vi "tm_preparecapture.vi"(8 "error in (no error)":errorcluster, 9 "Frames":i32, 10 "Capture mode":i32(ring) items=["Snap", "Sequence"], 11 "Handle in":u32) -> (0 "error out":errorcluster, 2 "Buffer":T1, 3 "Handle out":u32, 4 "Image type":u32)   [LabVIEW 2015]
uses:
  tmcamcon.dll
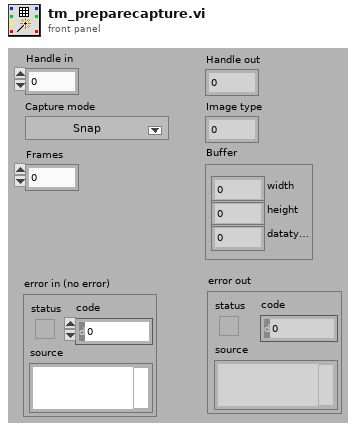
[diagram p1: front panel]
types:
  T1 = cluster{"width":u32, "height":u32, "datatype":u32}
  T2 = cluster{"height":u32, "width":u32, "datatype":u32}
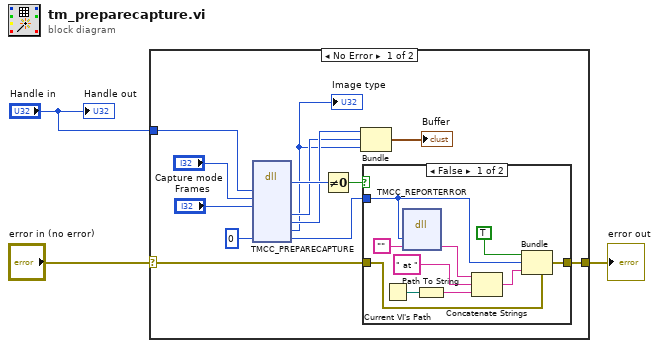
[diagram p0: block diagram]
diagram:
  n1 = case shown="No Error" "error in (no error)" {
    selector: "error in (no error)" -> [w11 w28]
    tunnel: [w10 w28] -> w1
    tunnel: "Handle in" -> [w15 _]
    frame No Error {
      n2 = dll-call lib="tmcamcon.dll" fn="TMCC_PREPARECAPTURE"("index"=w15, "mode"="Capture mode", "frames"="Frames", "Erval"=0) -> ("return type"=w16:u32, "width"=w6:u32, "height"=w7:u32, "datatype"=w5:u32, "Erval"=w12:i32)  [unwired: 9 in, 2 out]
      "Image type" <- w5
      n3 = Not Equal To 0?(x=w16) -> (x != 0?=w13:bool)
      n4 = Bundle("height"=w7, "width"=w6, "datatype"=w5) -> (→"Buffer":T2)  [unwired: 1 in]
      n5 = case shown="False" w13 {
        tunnel: w11 -> [w26 w27]
        tunnel: [w25 w27] -> w10
        tunnel: w12 -> [w19 _]
        frame False {
          n6 = Current VI's Path() -> (path=w24:path)
          n7 = dll-call lib="tmcamcon.dll" fn="TMCC_REPORTERROR"("error"=w19, "buf"="") -> ("buf"=w18:string)  [unwired: 5 in, 2 out]
          n8 = Path To String(path=w24) -> (string=w20:string)
          n9 = Concatenate Strings(w18, " at ", w20) -> (w23:string)
          n10 = Bundle(cluster=w26, "status"=TRUE, "code"=w19, "source"=w23) -> (w25:errorcluster)
        }
        frame True {
        }
      }
    }
    frame Error {
    }
  }
  "error out" <- w1
  "Handle out" <- "Handle in"
